vi "audio-stim.vi"() -> ()   [LabVIEW 2013]
panel:
  in  "stop":bool
  in  "Save Stimulus List":bool
  in  "Load Parameter List":bool
  in  "Save Parameter List":bool
  in  "Repetitions":i32=10 caption="# of Random Repetitions for Each Stimulus" min=2
  in  "Parameter List":dbl[][](array[numeric])=[[3.0, 200.0, 1.0, 500.0], [3.0, 200.0, 1.0, 1000.0]]
  out "Stimulus List":dbl[][](array[numeric])
  in  "Load Stimulus List":bool
  out "Stimulus List Path":path
  out "Parameter Path":path
  in  "Play":bool
  in  "Generate Stimulus List":bool
  # "Stim#, Stim Type, Duration, Amplitude, Param 1, Param 2, Param 3, Param 4"
  # "Stim Type, Duration, Amplitude, Param 1, Param 2, Param 3, Param 4"
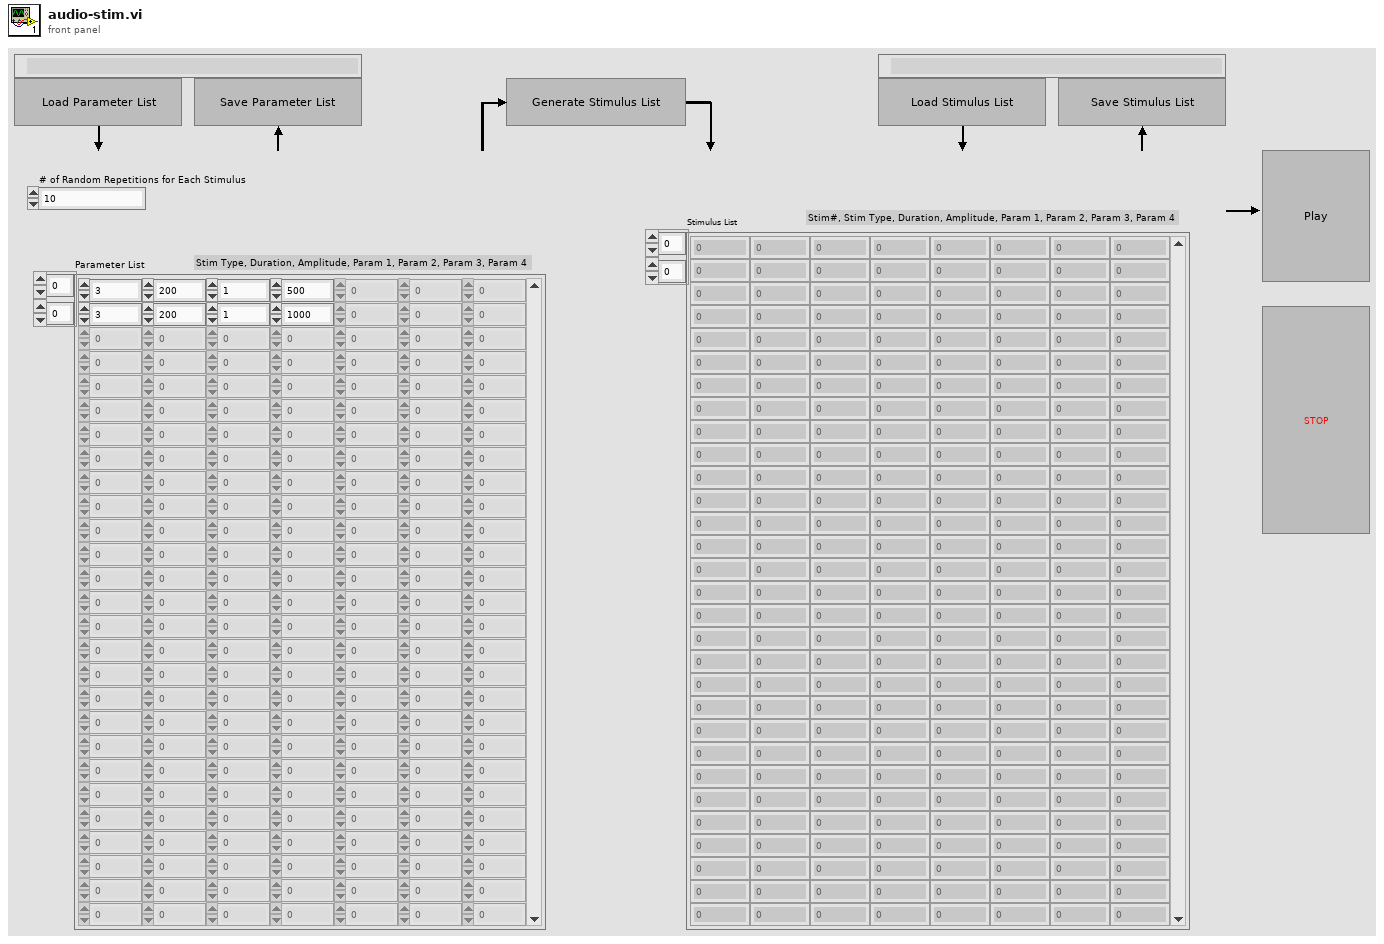
[diagram p1: front panel]
types:
  T1 = enum8{"Enabled", "Disabled", "Disabled and Grayed Out"}
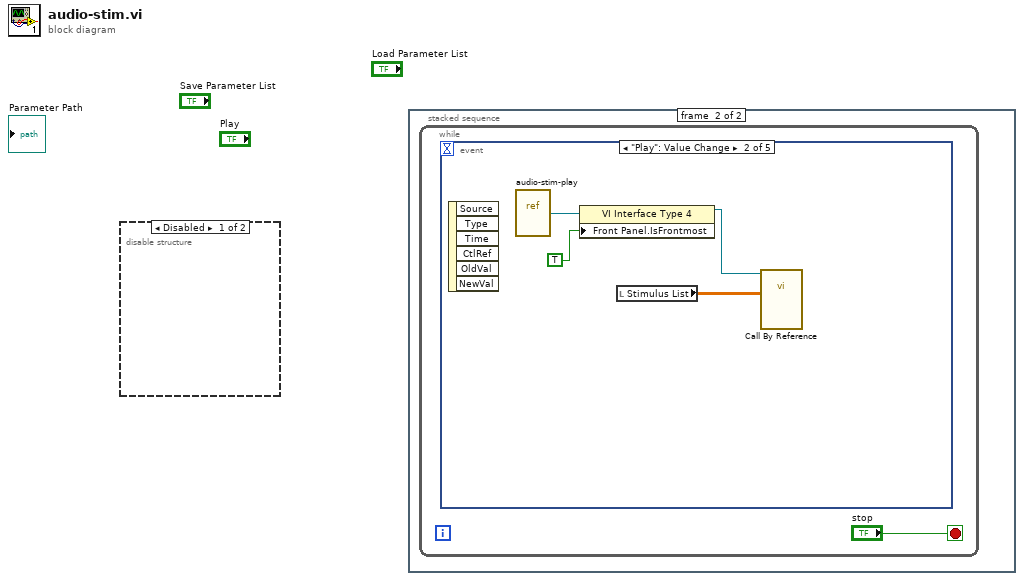
[diagram p0: block diagram]
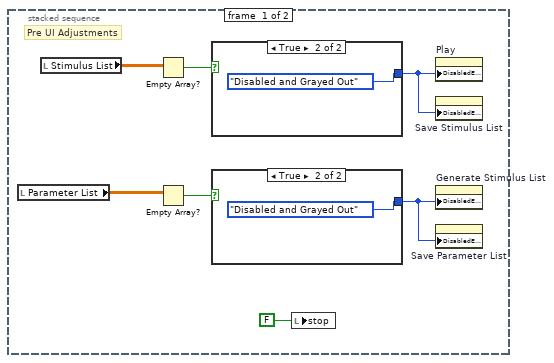
[diagram p3: hidden frame]
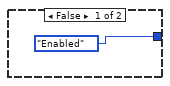
[diagram p4: hidden frame]
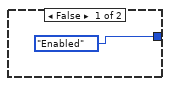
[diagram p5: hidden frame]
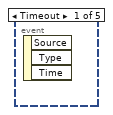
[diagram p6: hidden frame]
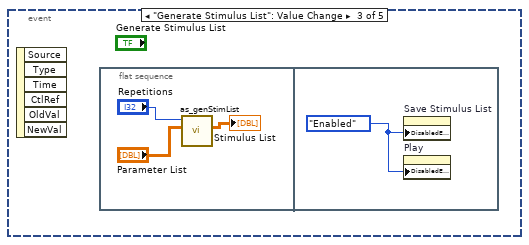
[diagram p7: hidden frame]
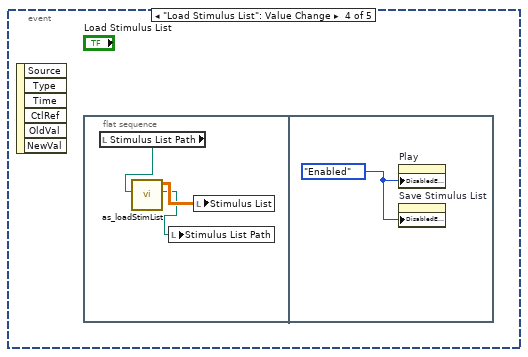
[diagram p8: hidden frame]
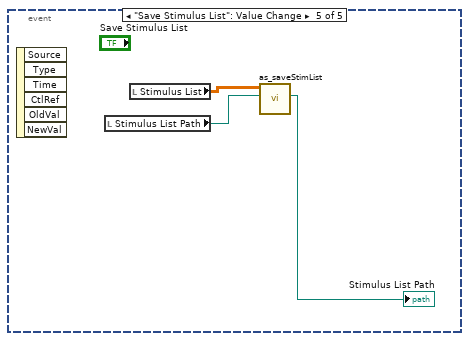
[diagram p9: hidden frame]
diagram:
  n1 = disable-structure shown="Disabled" {
    frame Disabled {
    }
    frame Enabled {
    }
  }
  n2 = stacked-sequence {
    frame #0 {
      # "Pre UI Adjustments"
      n3 = local read "Parameter List"() -> (w2:dbl[][])
      n4 = local read "Stimulus List"() -> (w7:dbl[][])
      n5 = Empty Array?(array=w7) -> (empty?=w6:bool)
      n6 = Empty Array?(array=w2) -> (empty?=w4:bool)
      n7 = case shown="True" w6 {
        tunnel: [T1."Enabled" ("Disabled") T1."Disabled and Grayed Out" ("Disabled")] -> w5
        frame False {
        }
        frame True {
        }
      }
      n8 = case shown="True" w4 {
        tunnel: [T1."Enabled" ("Disabled") T1."Disabled and Grayed Out" ("Disabled")] -> w3
        frame False {
        }
        frame True {
        }
      }
      n9 = local write "stop"(FALSE ("stop")) -> ()
      n10 = property on="Play" class="Bool (strict)"("DisabledEnum"=w5) -> ()  [unwired: 2 in, 2 out]
      n11 = property on="Save Stimulus List" class="Bool"("DisabledEnum"=w5) -> ()  [unwired: 2 in, 2 out]
      n12 = property on="Generate Stimulus List" class="Bool"("DisabledEnum"=w3) -> ()  [unwired: 2 in, 2 out]
      n13 = property on="Save Parameter List" class="Bool"("DisabledEnum"=w3) -> ()  [unwired: 2 in, 2 out]
    }
    frame #1 {
      n14 = while {
        stop <- "stop" stop-if-true
        n15 = event shown="[1] \"Play\": Value Change" {
          selector: _ -> [_ _ _ _ _]
          dyn-events: _ -> [_ _ _ _ _]
          timeout: _ -> [_ _ _ _ _]
          event Timeout {
            n16 = event-data() -> ()  [unwired: 1 in, 3 out]
          }
          event "Play": Value Change {
            n17 = event-data() -> ()  [unwired: 1 in, 6 out]
            n18 = vi-ref "audio-stim-play.vi"() -> (w16:refnum<vi>)
            n19 = property class="VI Interface Type 4"(reference=w16, "Front Panel.IsFrontmost"=TRUE ("Execution:Show Front Panel On Call")) -> (reference out=w13:refnum<vi>)  [unwired: 1 in, 1 out]
            n20 = local read "Stimulus List"() -> (w14:dbl[][])
            n21 = call-by-ref "?"(reference=w13, "Stimulus List"=w14) -> ()  [unwired: 12 in, 2 out]
          }
          event "Generate Stimulus List": Value Change {
            n22 = event-data() -> ()  [unwired: 1 in, 6 out]
            n23 = flat-sequence {
              frame #0 {
                n24 = call "as_genStimList.vi"("Stimulus Parameters"="Parameter List", "Repetitions"="Repetitions") -> ("Stimulus List"=→"Stimulus List":dbl[][])  [unwired: 9 in]
              }
              frame #1 {
                w20 = T1."Enabled" ("Disabled")
                n25 = property on="Save Stimulus List" class="Bool"("DisabledEnum"=w20) -> ()  [unwired: 2 in, 2 out]
                n26 = property on="Play" class="Bool (strict)"("DisabledEnum"=w20) -> ()  [unwired: 2 in, 2 out]
              }
            }
          }
          event "Load Stimulus List": Value Change {
            n27 = event-data() -> ()  [unwired: 1 in, 6 out]
            n28 = flat-sequence {
              frame #0 {
                n29 = local read "Stimulus List Path"() -> (w23:path)
                n30 = call "as_loadStimList.vi"("Path In"=w23) -> ("Path"=w21:path, "Stimulus List"=w22:dbl[][])  [unwired: 4 in, 1 out]
                n31 = local write "Stimulus List Path"(w21) -> ()
                n32 = local write "Stimulus List"(w22) -> ()
              }
              frame #1 {
                w24 = T1."Enabled" ("Disabled")
                n33 = property on="Play" class="Bool (strict)"("DisabledEnum"=w24) -> ()  [unwired: 2 in, 2 out]
                n34 = property on="Save Stimulus List" class="Bool"("DisabledEnum"=w24) -> ()  [unwired: 2 in, 2 out]
              }
            }
          }
          event "Save Stimulus List": Value Change {
            n35 = event-data() -> ()  [unwired: 1 in, 6 out]
            n36 = local read "Stimulus List Path"() -> (w26:path)
            n37 = local read "Stimulus List"() -> (w27:dbl[][])
            n38 = call "as_saveStimList.vi"("Path In"=w26, "Stimulus List"=w27) -> ("Path"=→"Stimulus List Path":path)  [unwired: 4 in, 1 out]
          }
        }
      }
    }
  }
